vi "Monitor-NewScanSizeAndOffset.vi"(6 "um/px":cluster{" um/px X":dbl, "um/px Y":dbl}, 7 "Zoom Rect coords px":T2, 9 "Scan Size Center pixels":T3) -> (1 "Zoom Center coords um":T1, 4 "New Scan Size":cluster{"Width um":dbl, " Height um":dbl})   [LabVIEW 2016]
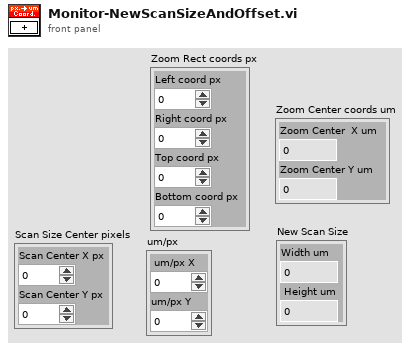
[diagram p1: front panel]
types:
  T1 = cluster{"Zoom Center  X um":dbl, "Zoom Center Y um":dbl}
  T2 = cluster{"Left coord px":dbl, "Right coord px":dbl, "Top coord px":dbl, "Bottom coord px":dbl}
  T3 = cluster{"Scan Center X px":dbl, "Scan Center Y px":dbl}
  T4 = cluster{"Left coord px":dbl, "Right coord px":dbl}
  T5 = cluster{"Top coord px":dbl, "Bottom coord px":dbl}
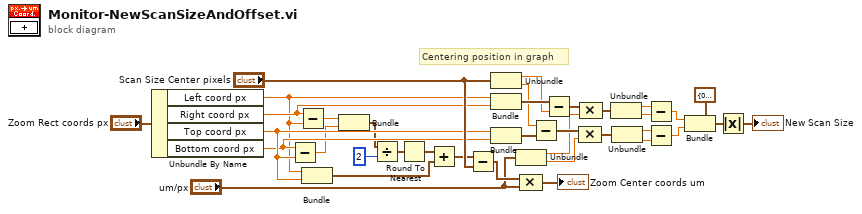
[diagram p0: block diagram]
diagram:
  # "Centering position in graph"
  n1 = Unbundle By Name("Zoom Rect coords px") -> ("Left coord px"=w8:dbl, "Right coord px"=w10:dbl, "Top coord px"=w11:dbl, "Bottom coord px"=w9:dbl)
  n2 = Subtract ("Height")(x=w9, y=w11) -> (x-y=w3:dbl)
  n3 = Subtract ("Width")(x=w10, y=w8) -> (x-y=w16:dbl)
  n4 = Bundle("Left coord px"=w8, "Top coord px"=w11) -> (w17:cluster{"Left coord px":dbl, "Top coord px":dbl})  [unwired: 1 in]
  n5 = Bundle(w16, w3) -> (w4:cluster{dbl, dbl})  [unwired: 1 in]
  n6 = Divide(x=w4, y=i16 2) -> (x/y=w13:cluster{dbl, dbl})
  n7 = Round To Nearest(number=w13) -> (nearest integer value=w15:cluster{dbl, dbl})
  n8 = Add(x=w15, y=w17) -> (x+y=w12:cluster{dbl, dbl})
  n9 = Subtract(x=w12, y="Scan Size Center pixels") -> (x-y=w2:cluster{dbl, dbl})
  n10 = Unbundle("Scan Size Center pixels") -> ("Scan Center X px"=w6:dbl, "Scan Center Y px"=w5:dbl)
  n11 = Bundle("Left coord px"=w8, "Right coord px"=w10) -> (w29:T4)  [unwired: 1 in]
  n12 = Bundle("Top coord px"=w11, "Bottom coord px"=w9) -> (w34:T5)  [unwired: 1 in]
  n13 = Unbundle("um/px") -> ("um/px X"=w7:dbl, "um/px Y"=w18:dbl)
  n14 = Compound Arithmetic op=MULTIPLY(w2, "um/px") -> (→"Zoom Center coords um":cluster{dbl, dbl})
  n15 = Subtract(x=w5, y=w34) -> (x-y=w33:T5)
  n16 = Subtract(x=w29, y=w6) -> (x-y=w28:T4)
  n17 = Compound Arithmetic op=MULTIPLY(w33, w18) -> (w32:T5)
  n18 = Compound Arithmetic op=MULTIPLY(w28, w7) -> (w27:T4)
  n19 = Unbundle(w27) -> ("Left coord px"=w26:dbl, "Right coord px"=w25:dbl)
  n20 = Unbundle(w32) -> ("Top coord px"=w31:dbl, "Bottom coord px"=w30:dbl)
  n21 = Subtract(x=w26, y=w25) -> (x-y=w24:dbl)
  n22 = Subtract(x=w31, y=w30) -> (x-y=w23:dbl)
  n23 = Bundle(cluster=cluster{"Width um":dbl, " Height um":dbl} {"Width um"=0.0, " Height um"=0.0} ("New Scan Size um"), "Width um"=w24, "Height um"=w23) -> (w22:cluster{"Width um":dbl, " Height um":dbl})
  n24 = Absolute Value(x=w22) -> (abs(x)=→"New Scan Size":cluster{"Width um":dbl, " Height um":dbl})
